vi "TimeCount1.vi"(1 "start":bool, 2 "reset":bool) -> (0 "time":dbl)   [LabVIEW 2014]
panel:
  out "stateClock":enum16{"reset", "start", "stop"}(ring)
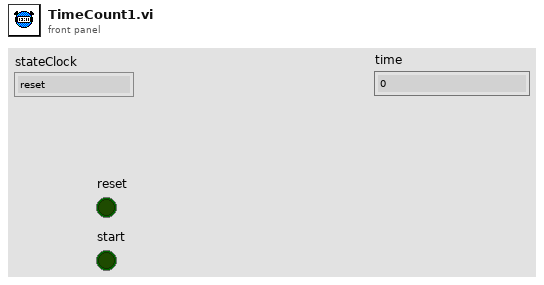
[diagram p1: front panel]
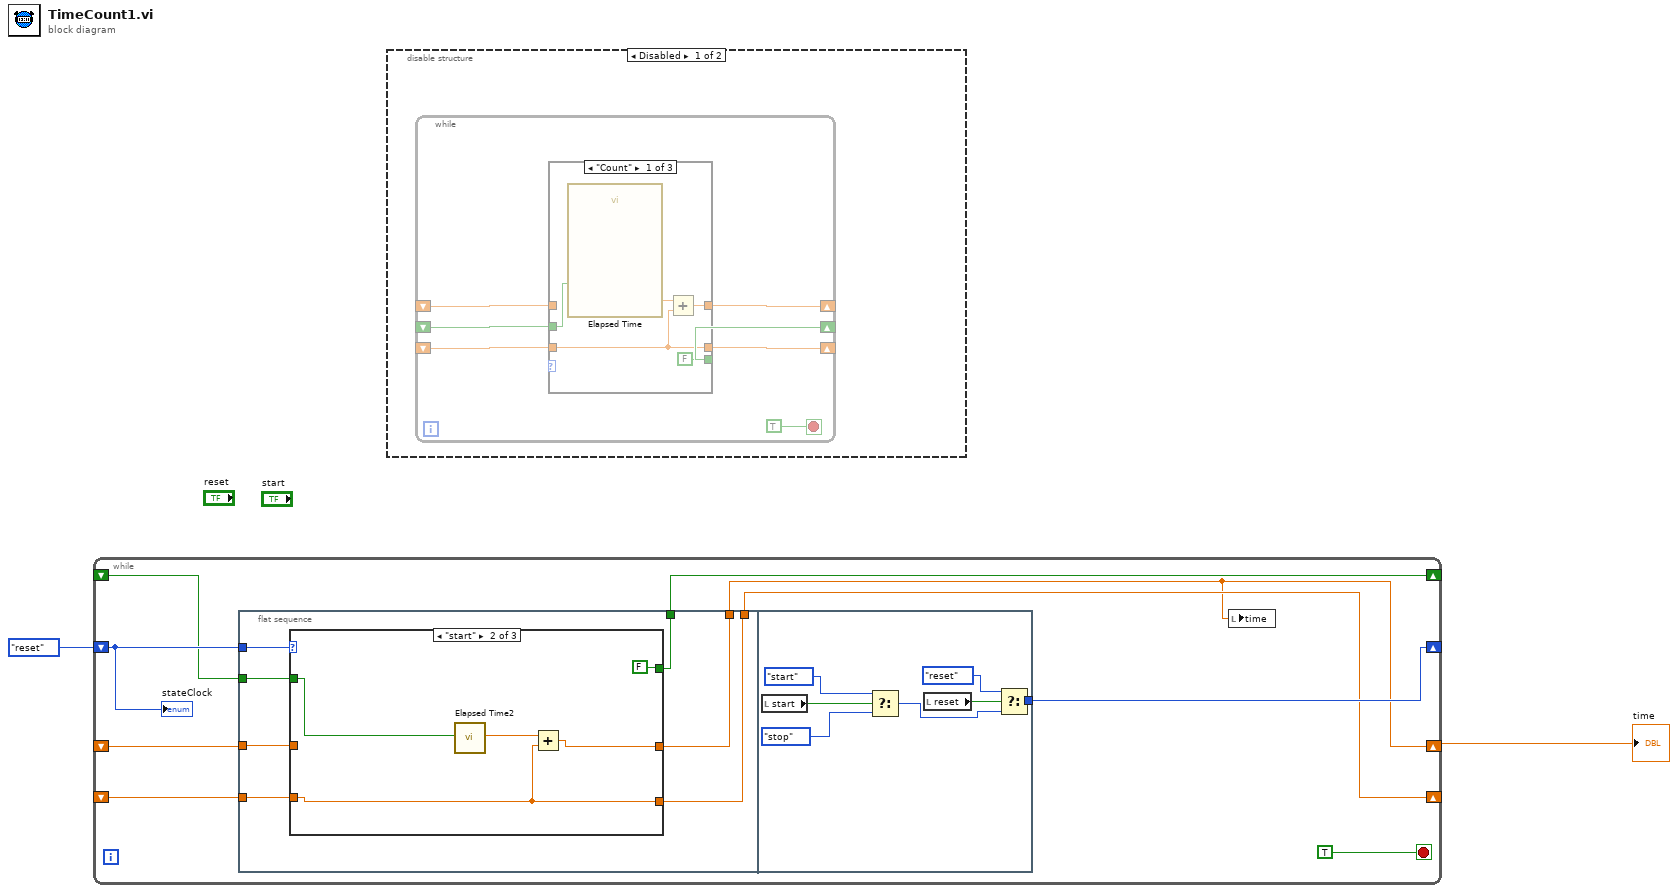
[diagram p0: block diagram]
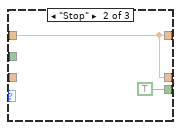
[diagram p2: hidden frame]
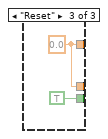
[diagram p3: hidden frame]
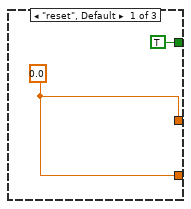
[diagram p5: hidden frame]
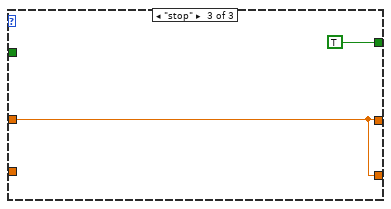
[diagram p6: hidden frame]
diagram:
  n1 = while {
    shift-right: [w10] -> _
    shift-left: enum16{"reset", "start", "stop"}."reset" ("stateClock") -> [w11]
    shift-right: [w6] -> w1
    shift-left: _ -> [w9]
    shift-right: [w8] -> _
    shift-left: _ -> [w7]
    shift-right: [w5] -> _
    shift-left: _ -> [w4]
    stop <- TRUE stop-if-true
    n2 = flat-sequence {
      tunnel: w11 -> [w18]
      tunnel: [w16] -> w6
      tunnel: w9 -> [w17]
      tunnel: [w15] -> w8
      tunnel: w7 -> [w14]
      tunnel: [w13] -> w5
      tunnel: w4 -> [w12]
      tunnel: [w28] -> w10
      frame #0 {
        n3 = case shown="\"start\"" w18 {
          tunnel: [w20 w23 w27] -> w16
          tunnel: w17 -> [_ _ w27]
          tunnel: [w20 w24 w27] -> w15
          tunnel: w14 -> [_ w24 _]
          tunnel: [TRUE FALSE TRUE] -> w13
          tunnel: w12 -> [_ w21 _]
          frame "reset", Default {
            w20 = 0.0
          }
          frame "start" {
            n4 = call "Elapsed Time2"("Reset"=w21) -> ("Elapsed Time (s)"=w25:dbl)  [unwired: 11 in, 7 out]
            n5 = Add(x=w25, y=w24) -> (x+y=w23:dbl)
          }
          frame "stop" {
          }
        }
      }
      frame #1 {
        n6 = local read "start"() -> (w31:bool)
        n7 = Select(t=enum16{"reset", "start", "stop"}."start" ("stateClock"), s=w31, f=enum16{"reset", "start", "stop"}."stop" ("stateClock")) -> (s? t:f=w34:enum16{"reset", "start", "stop"})
        n8 = local read "reset"() -> (w32:bool)
        n9 = Select(t=enum16{"reset", "start", "stop"}."reset" ("stateClock"), s=w32, f=w34) -> (s? t:f=w28:enum16{"reset", "start", "stop"})
      }
    }
    n10 = local write "time"(w6) -> ()
    "stateClock" <- w11
  }
  "time" <- w1
  n11 = disable-structure shown="Disabled" {
    frame Disabled {
      n12 = while {
        shift-right: [w41] -> _
        shift-left: _ -> [w40]
        shift-right: [w37] -> _
        shift-left: _ -> [w38]
        shift-right: [w35] -> _
        shift-left: _ -> [w36]
        stop <- TRUE stop-if-true
        n13 = case shown="\"Count\"" {
          selector: _ -> [_ _ _]
          tunnel: [w44 w47 w49] -> w41
          tunnel: w40 -> [_ w47 _]
          tunnel: w38 -> [w45 _ _]
          tunnel: [FALSE TRUE TRUE] -> w37
          tunnel: w36 -> [w43 _ _]
          tunnel: [w43 w47 w49] -> w35
          frame "Count" {
            n14 = call "Elapsed Time"("Reset"=w45) -> ("Elapsed Time (s)"=w46:dbl)  [unwired: 11 in, 7 out]
            n15 = Add(x=w46, y=w43) -> (x+y=w44:dbl)
          }
          frame "Stop" {
          }
          frame "Reset" {
            w49 = 0.0 ("Elapsed Time (s)")
          }
        }
      }
    }
    frame Enabled {
    }
  }
